vi "SeCrTs-Data queue.vi"(3 "error in":errorcluster) -> (7 "Data FIFO Ref":T1, 10 "error out":errorcluster)   [LabVIEW 2022 SP3]
uses:
  RT Controls/SeCrTs-Data FIFO.ctl
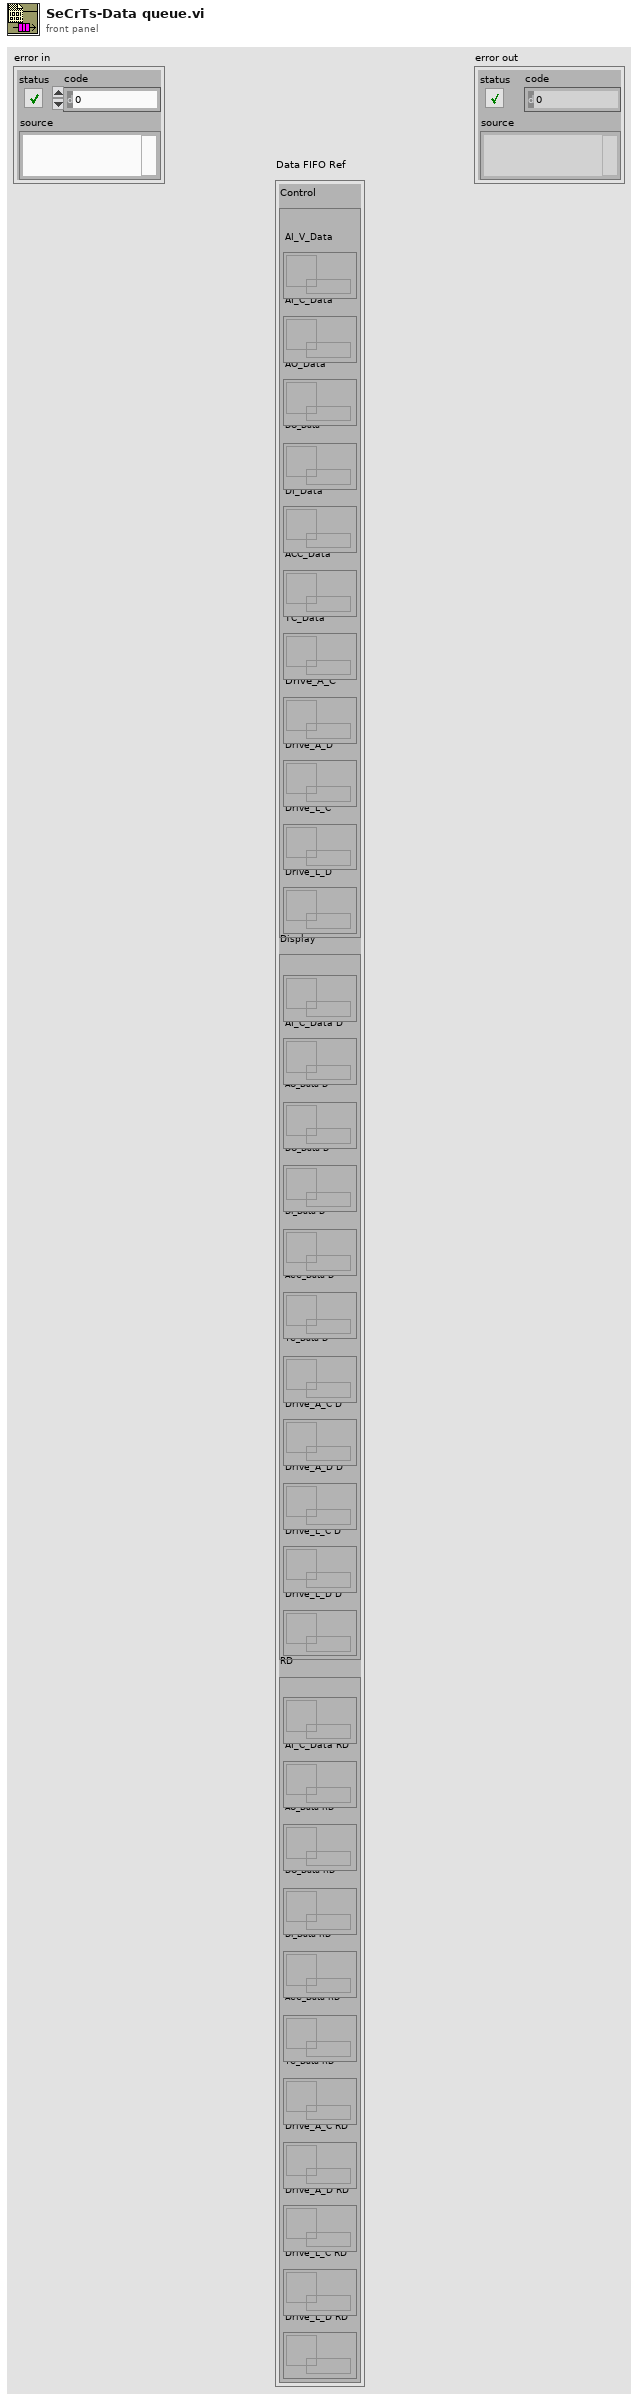
[diagram p1: front panel]
types:
  T1 = typedef "SeCrTs-Data FIFO.ctl" = cluster{"Control":cluster{"AI_V_Data":refnum<queue>, "AI_C_Data":refnum<queue>, "AO_Data":refnum<queue>, "DO_Data":refnum<queue>, "DI_Data":refnum<queue>, "ACC_Data":refnum<queue>, "TC_Data":refnum<queue>, "Drive_A_C":refnum<queue>, "Drive_A_D":refnum<queue>, "Drive_L_C":refnum<queue>, "Drive_L_D":refnum<queue>}, "Display":cluster{"AI_V_Data D":refnum<queue>, "AI_C_Data D":refnum<queue>, "AO_Data D":refnum<queue>, "DO_Data D":refnum<queue>, "DI_Data D":refnum<queue>, "ACC_Data D":refnum<queue>, "TC_Data D":refnum<queue>, "Drive_A_C D":refnum<queue>, "Drive_A_D D":refnum<queue>, "Drive_L_C D":refnum<queue>, "Drive_L_D D":refnum<queue>}, "RD":cluster{"AI_V_Data RD":refnum<queue>, "AI_C_Data RD":refnum<queue>, "AO_Data RD":refnum<queue>, "DO_Data RD":refnum<queue>, "DI_Data RD":refnum<queue>, "ACC_Data RD":refnum<queue>, "TC_Data RD":refnum<queue>, "Drive_A_C RD":refnum<queue>, "Drive_A_D RD":refnum<queue>, "Drive_L_C RD":refnum<queue>, "Drive_L_D RD":refnum<queue>}}
  T2 = cluster{"AI_V_Data D":refnum<queue>, "AI_C_Data D":refnum<queue>, "AO_Data D":refnum<queue>, "DO_Data D":refnum<queue>, "DI_Data D":refnum<queue>, "ACC_Data D":refnum<queue>, "TC_Data D":refnum<queue>, "Drive_A_C D":refnum<queue>, "Drive_A_D D":refnum<queue>, "Drive_L_C D":refnum<queue>, "Drive_L_D D":refnum<queue>}
  T3 = cluster{"AI_V_Data":refnum<queue>, "AI_C_Data":refnum<queue>, "AO_Data":refnum<queue>, "DO_Data":refnum<queue>, "DI_Data":refnum<queue>, "ACC_Data":refnum<queue>, "TC_Data":refnum<queue>, "Drive_A_C":refnum<queue>, "Drive_A_D":refnum<queue>, "Drive_L_C":refnum<queue>, "Drive_L_D":refnum<queue>}
  T4 = cluster{"AI_V_Data RD":refnum<queue>, "AI_C_Data RD":refnum<queue>, "AO_Data RD":refnum<queue>, "DO_Data RD":refnum<queue>, "DI_Data RD":refnum<queue>, "ACC_Data RD":refnum<queue>, "TC_Data RD":refnum<queue>, "Drive_A_C RD":refnum<queue>, "Drive_A_D RD":refnum<queue>, "Drive_L_C RD":refnum<queue>, "Drive_L_D RD":refnum<queue>}
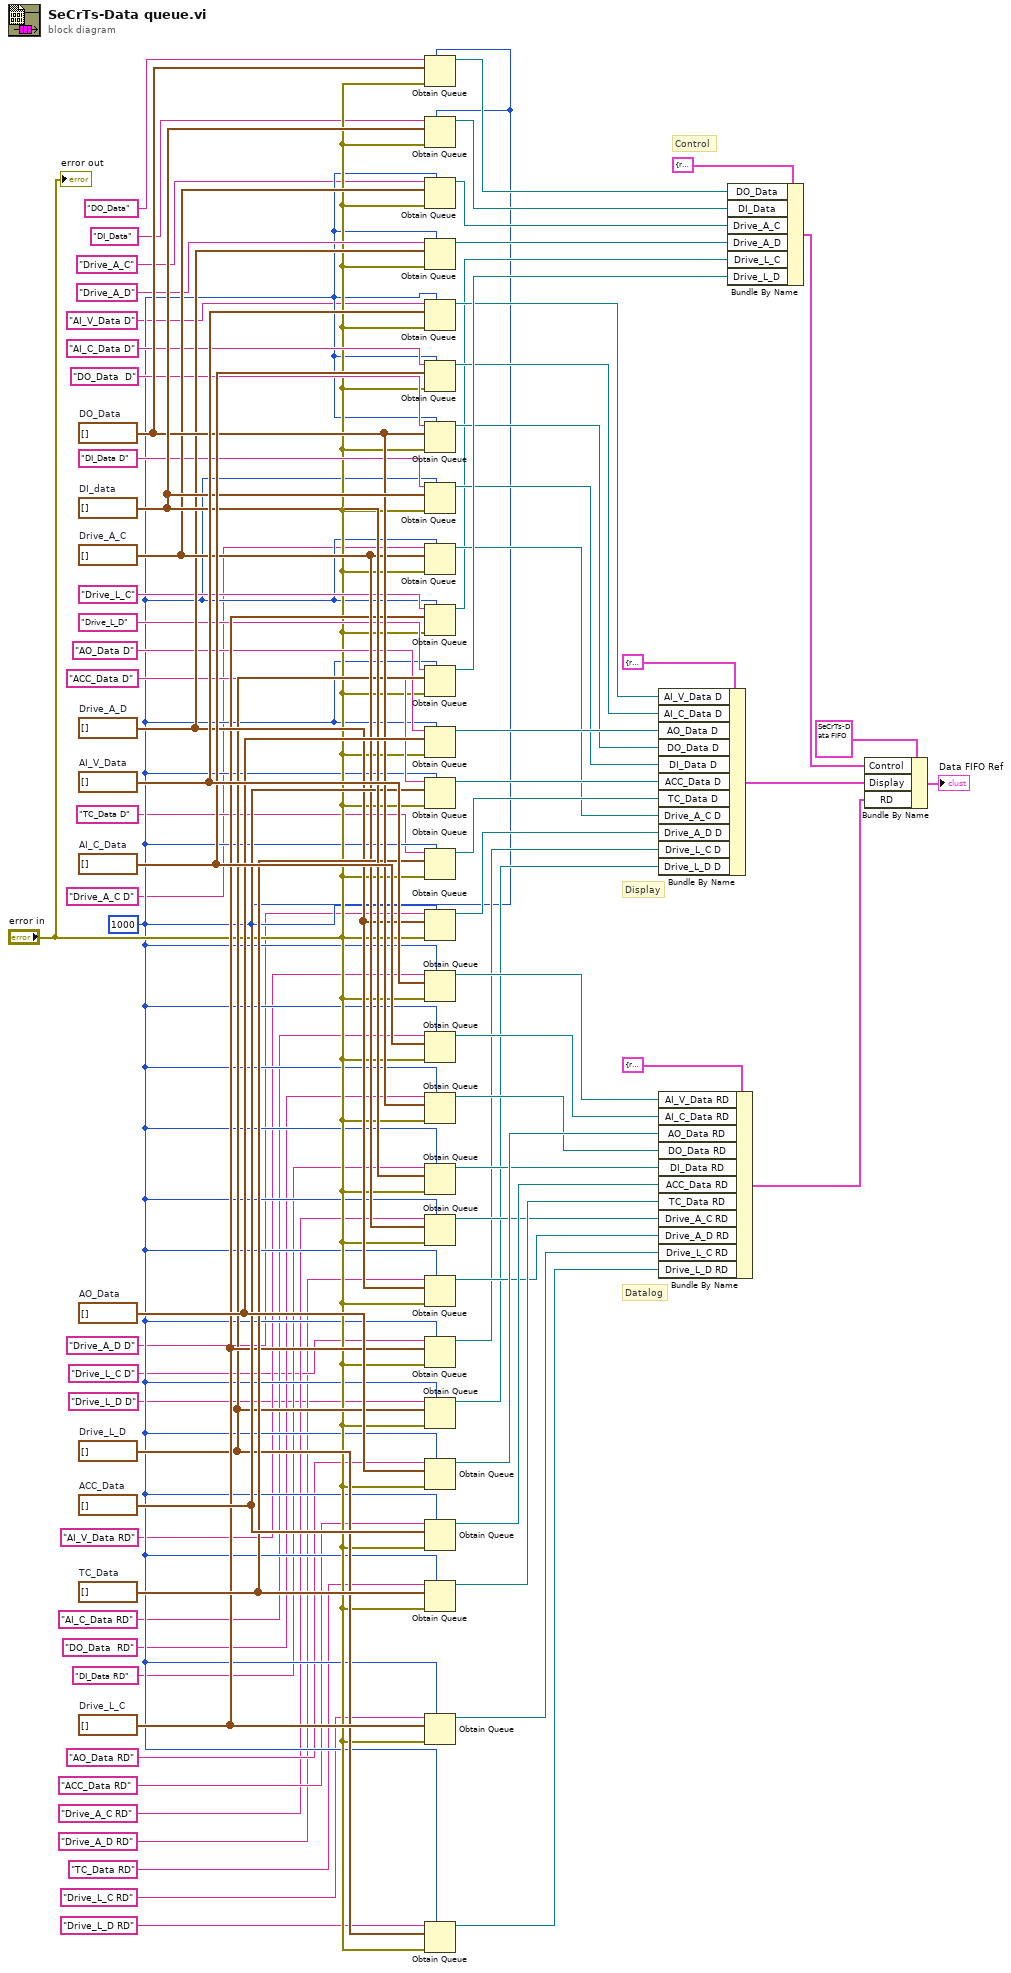
[diagram p0: block diagram]
diagram:
  w23 = 1000 ("max queue size (-1, unlimited)")
  w77 = waveform(dbl)[] []  # AI_V_Data
  w67 = waveform(dbl)[] []  # Drive_L_D
  w68 = waveform(dbl)[] []  # Drive_L_C
  w69 = waveform(dbl)[] []  # Drive_A_D
  w70 = waveform(dbl)[] []  # Drive_A_C
  w71 = waveform(dbl)[] []  # TC_Data
  w72 = waveform(dbl)[] []  # ACC_Data
  w74 = digitalwaveform[] []  # DI_data
  w73 = waveform(dbl)[] []  # DO_Data
  w75 = waveform(dbl)[] []  # AO_Data
  w76 = waveform(dbl)[] []  # AI_C_Data
  # "Datalog"
  # "Display"
  # "Control"
  n1 = Obtain Queue(max queue size (-1, unlimited)=w23, name (unnamed)="DO_Data", element data type=w73, error in (no error)="error in") -> (queue out=w45:refnum<queue>)  [unwired: 1 in, 2 out]
  n2 = Obtain Queue(max queue size (-1, unlimited)=w23, name (unnamed)="DI_Data", element data type=w74, error in (no error)="error in") -> (queue out=w44:refnum<queue>)  [unwired: 1 in, 2 out]
  n3 = Obtain Queue(max queue size (-1, unlimited)=w23, name (unnamed)="Drive_A_C", element data type=w70, error in (no error)="error in") -> (queue out=w43:refnum<queue>)  [unwired: 1 in, 2 out]
  n4 = Obtain Queue(max queue size (-1, unlimited)=w23, name (unnamed)="Drive_A_D", element data type=w69, error in (no error)="error in") -> (queue out=w42:refnum<queue>)  [unwired: 1 in, 2 out]
  n5 = Obtain Queue(max queue size (-1, unlimited)=w23, name (unnamed)="AI_V_Data D", element data type=w77, error in (no error)="error in") -> (queue out=w39:refnum<queue>)  [unwired: 1 in, 2 out]
  n6 = Obtain Queue(max queue size (-1, unlimited)=w23, name (unnamed)="AI_C_Data D", element data type=w76, error in (no error)="error in") -> (queue out=w38:refnum<queue>)  [unwired: 1 in, 2 out]
  n7 = Obtain Queue(max queue size (-1, unlimited)=w23, name (unnamed)="DO_Data  D", element data type=w73, error in (no error)="error in") -> (queue out=w36:refnum<queue>)  [unwired: 1 in, 2 out]
  n8 = Obtain Queue(max queue size (-1, unlimited)=w23, name (unnamed)="DI_Data D", element data type=w74, error in (no error)="error in") -> (queue out=w35:refnum<queue>)  [unwired: 1 in, 2 out]
  n9 = Obtain Queue(max queue size (-1, unlimited)=w23, name (unnamed)="Drive_A_C D", element data type=w70, error in (no error)="error in") -> (queue out=w32:refnum<queue>)  [unwired: 1 in, 2 out]
  n10 = Obtain Queue(max queue size (-1, unlimited)=w23, name (unnamed)="Drive_L_C", element data type=w68, error in (no error)="error in") -> (queue out=w24:refnum<queue>)  [unwired: 1 in, 2 out]
  n11 = Obtain Queue(max queue size (-1, unlimited)=w23, name (unnamed)="Drive_L_D", element data type=w67, error in (no error)="error in") -> (queue out=w41:refnum<queue>)  [unwired: 1 in, 2 out]
  n12 = Obtain Queue(max queue size (-1, unlimited)=w23, name (unnamed)="AO_Data D", element data type=w75, error in (no error)="error in") -> (queue out=w37:refnum<queue>)  [unwired: 1 in, 2 out]
  n13 = Obtain Queue(max queue size (-1, unlimited)=w23, name (unnamed)="ACC_Data D", element data type=w72, error in (no error)="error in") -> (queue out=w34:refnum<queue>)  [unwired: 1 in, 2 out]
  n14 = Obtain Queue(max queue size (-1, unlimited)=w23, name (unnamed)="TC_Data D", element data type=w71, error in (no error)="error in") -> (queue out=w33:refnum<queue>)  [unwired: 1 in, 2 out]
  n15 = Obtain Queue(max queue size (-1, unlimited)=w23, name (unnamed)="Drive_A_D D", element data type=w69, error in (no error)="error in") -> (queue out=w31:refnum<queue>)  [unwired: 1 in, 2 out]
  n16 = Obtain Queue(max queue size (-1, unlimited)=w23, name (unnamed)="AI_V_Data RD", element data type=w77, error in (no error)="error in") -> (queue out=w58:refnum<queue>)  [unwired: 1 in, 2 out]
  n17 = Obtain Queue(max queue size (-1, unlimited)=w23, name (unnamed)="AI_C_Data RD", element data type=w76, error in (no error)="error in") -> (queue out=w56:refnum<queue>)  [unwired: 1 in, 2 out]
  n18 = Obtain Queue(max queue size (-1, unlimited)=w23, name (unnamed)="DO_Data  RD", element data type=w73, error in (no error)="error in") -> (queue out=w54:refnum<queue>)  [unwired: 1 in, 2 out]
  n19 = Obtain Queue(max queue size (-1, unlimited)=w23, name (unnamed)="DI_Data RD", element data type=w74, error in (no error)="error in") -> (queue out=w53:refnum<queue>)  [unwired: 1 in, 2 out]
  n20 = Obtain Queue(max queue size (-1, unlimited)=w23, name (unnamed)="Drive_A_C RD", element data type=w70, error in (no error)="error in") -> (queue out=w50:refnum<queue>)  [unwired: 1 in, 2 out]
  n21 = Obtain Queue(max queue size (-1, unlimited)=w23, name (unnamed)="Drive_A_D RD", element data type=w69, error in (no error)="error in") -> (queue out=w49:refnum<queue>)  [unwired: 1 in, 2 out]
  n22 = Obtain Queue(max queue size (-1, unlimited)=w23, name (unnamed)="Drive_L_C D", element data type=w68, error in (no error)="error in") -> (queue out=w30:refnum<queue>)  [unwired: 1 in, 2 out]
  n23 = Obtain Queue(max queue size (-1, unlimited)=w23, name (unnamed)="Drive_L_D D", element data type=w67, error in (no error)="error in") -> (queue out=w29:refnum<queue>)  [unwired: 1 in, 2 out]
  n24 = Obtain Queue(max queue size (-1, unlimited)=w23, name (unnamed)="AO_Data RD", element data type=w75, error in (no error)="error in") -> (queue out=w55:refnum<queue>)  [unwired: 1 in, 2 out]
  n25 = Obtain Queue(max queue size (-1, unlimited)=w23, name (unnamed)="ACC_Data RD", element data type=w72, error in (no error)="error in") -> (queue out=w52:refnum<queue>)  [unwired: 1 in, 2 out]
  n26 = Obtain Queue(max queue size (-1, unlimited)=w23, name (unnamed)="TC_Data RD", element data type=w71, error in (no error)="error in") -> (queue out=w51:refnum<queue>)  [unwired: 1 in, 2 out]
  n27 = Obtain Queue(max queue size (-1, unlimited)=w23, name (unnamed)="Drive_L_C RD", element data type=w68, error in (no error)="error in") -> (queue out=w48:refnum<queue>)  [unwired: 1 in, 2 out]
  n28 = Obtain Queue(max queue size (-1, unlimited)=w23, name (unnamed)="Drive_L_D RD", element data type=w67, error in (no error)="error in") -> (queue out=w47:refnum<queue>)  [unwired: 1 in, 2 out]
  n29 = Bundle By Name(cluster=T2 {"AI_V_Data D"=refnum, "AI_C_Data D"=refnum, "AO_Data D"=refnum, "DO_Data D"=refnum, "DI_Data D"=refnum, "ACC_Data D"=refnum, "TC_Data D"=refnum, "Drive_A_C D"=refnum, "Drive_A_D D"=refnum, "Drive_L_C D"=refnum, "Drive_L_D D"=refnum}, "AI_V_Data D"=w39, "AI_C_Data D"=w38, "AO_Data D"=w37, "DO_Data D"=w36, "DI_Data D"=w35, "ACC_Data D"=w34, "TC_Data D"=w33, "Drive_A_C D"=w32, "Drive_A_D D"=w31, "Drive_L_C D"=w30, "Drive_L_D D"=w29) -> (w27:T2)
  n30 = Bundle By Name(cluster=T4 {"AI_V_Data RD"=refnum, "AI_C_Data RD"=refnum, "AO_Data RD"=refnum, "DO_Data RD"=refnum, "DI_Data RD"=refnum, "ACC_Data RD"=refnum, "TC_Data RD"=refnum, "Drive_A_C RD"=refnum, "Drive_A_D RD"=refnum, "Drive_L_C RD"=refnum, "Drive_L_D RD"=refnum}, "AI_V_Data RD"=w58, "AI_C_Data RD"=w56, "AO_Data RD"=w55, "DO_Data RD"=w54, "DI_Data RD"=w53, "ACC_Data RD"=w52, "TC_Data RD"=w51, "Drive_A_C RD"=w50, "Drive_A_D RD"=w49, "Drive_L_C RD"=w48, "Drive_L_D RD"=w47) -> (w26:T4)
  n31 = Bundle By Name(cluster=T3 {"AI_V_Data"=refnum, "AI_C_Data"=refnum, "AO_Data"=refnum, "DO_Data"=refnum, "DI_Data"=refnum, "ACC_Data"=refnum, "TC_Data"=refnum, "Drive_A_C"=refnum, "Drive_A_D"=refnum, "Drive_L_C"=refnum, "Drive_L_D"=refnum}, "DO_Data"=w45, "DI_Data"=w44, "Drive_A_C"=w43, "Drive_A_D"=w42, "Drive_L_C"=w24, "Drive_L_D"=w41) -> (w28:T3)
  n32 = Bundle By Name(cluster=T1 {"Control"={"AI_V_Data"=refnum, "AI_C_Data"=refnum, "AO_Data"=refnum, "DO_Data"=refnum, "DI_Data"=refnum, "ACC_Data"=refnum, "TC_Data"=refnum, "Drive_A_C"=refnum, "Drive_A_D"=refnum, "Drive_L_C"=refnum, "Drive_L_D"=refnum}, "Display"={"AI_V_Data D"=refnum, "AI_C_Data D"=refnum, "AO_Data D"=refnum, "DO_Data D"=refnum, "DI_Data D"=refnum, "ACC_Data D"=refnum, "TC_Data D"=refnum, "Drive_A_C D"=refnum, "Drive_A_D D"=refnum, "Drive_L_C D"=refnum, "Drive_L_D D"=refnum}, "RD"={"AI_V_Data RD"=refnum, "AI_C_Data RD"=refnum, "AO_Data RD"=refnum, "DO_Data RD"=refnum, "DI_Data RD"=refnum, "ACC_Data RD"=refnum, "TC_Data RD"=refnum, "Drive_A_C RD"=refnum, "Drive_A_D RD"=refnum, "Drive_L_C RD"=refnum, "Drive_L_D RD"=refnum}} ("Data FIFO Ref"), "Control"=w28, "Display"=w27, "RD"=w26) -> (→"Data FIFO Ref":T1)
  "error out" <- "error in"
